vi "Begin.vi"(8 "error in":errorcluster) -> (0 "error out":errorcluster)   [LabVIEW 2020]
doc: "Called before other user functions, this VI is expected to open initial I/O refnums, load in file data, and do all program initialization. Notice that the <B>error out</B> terminal is simply used for data flow. Wiring it to other structures or subVIs ensures that this VI runs first."
uses:
  <vilib>/Rock Robotics/WPI/DriverStation/WPI_DriverStationRobotMode2.ctl
  <vilib>/Rock Robotics/WPI/Joystick/WPI_JoystickDeviceEnum.ctl
  <vilib>/Rock Robotics/WPI/SafetyOutput/WPI_SafetyOutputConfigMenu.ctl
  <vilib>/Rock Robotics/SystemInterfaces/DIO/FPGA_DIOPWMChannel.ctl
  <vilib>/Rock Robotics/WPI/RobotDrive/WPI_RobotDriveDevRef.ctl
  <vilib>/Rock Robotics/WPI/MotorControl/WPI_MotorControlDeviceRef.ctl
  <vilib>/Rock Robotics/WPI/MotorControl/WPI_MotorControlType.ctl
  <vilib>/Rock Robotics/WPI/PWM/WPI_PWMDeadband.ctl
  <vilib>/Rock Robotics/SystemInterfaces/DIO/FPGA_DIOChannel.ctl
  <vilib>/Rock Robotics/WPI/Solenoid/WPI_SolenoidChannel.ctl
  <vilib>/Rock Robotics/WPI/Compressor/WPI_CompressorFeedbackMode.ctl
  <vilib>/Rock Robotics/SystemInterfaces/spilib/spi_bus.ctl
  Robot Global Data.vi
  <vilib>/Rock Robotics/Network Tables/NT Write String Array.vi
  <vilib>/Rock Robotics/WPI/Solenoid/WPI_SolenoidOpenDouble.vi
  <vilib>/Rock Robotics/WPI/Utilities/WPI_GetSetVariantRefNum.vi
  <vilib>/Rock Robotics/WPI/MotorControl/WPI_MotorControlOpen SPARK_MAX.vi
  <vilib>/Rock Robotics/WPI/Gyro/WPI_GyroXRS450_SPI_Open.vi
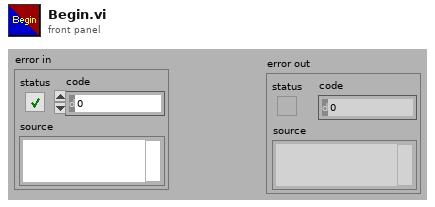
[diagram p1: front panel]
types:
  T1 = typedef "WPI_SolenoidChannel.ctl" = enum8{"Solenoid 0", "Solenoid 1", "Solenoid 2", "Solenoid 3", "Solenoid 4", "Solenoid 5", "Solenoid 6", "Solenoid 7", "Solenoid 8", "Solenoid 9", "Solenoid 10", "Solenoid 11", "Solenoid 12", "Solenoid 13", "Solenoid 14", "Solenoid 15", "Invalid"}
  T2 = typedef "spi_bus.ctl" = enum16{"SPI On-Board, CS0", "SPI On-Board, CS1", "SPI On-Board, CS2", "SPI On-Board, CS3", "SPI MXP", "Invalid"}
  T3 = typedef "WPI_CompressorFeedbackMode.ctl" = enum16{"Analog Only", "Digital Only", "Hybrid"}
  T4 = cluster{"Feedback Sensor":T3, "Max Pressure (PSI)":dbl, "Min Pressure (PSI)":dbl}
  T5 = typedef "WPI_JoystickDeviceEnum.ctl" = enum16{"USB 0", "USB 1", "USB 2", "USB 3", "USB 4", "USB 5"}
  T6 = typedef "WPI_RobotDriveDevRef.ctl" = cluster{"DevStatus":errorcluster, "Motors[]":T7[], "Square Inputs":bool, "Max Output":dbl}
  T7 = typedef "WPI_MotorControlDeviceRef.ctl" = cluster{"DeviceStatus":errorcluster, "Type":T8, "PWM":cluster{"PWM Channel":T9, "DeadBand":T10}, "CAN":cluster{"Device Number":u8, "SetOutput VI Ref":variant, "GetOutput VI Ref":variant, "Enable VI Ref":variant, "Disable VI Ref":variant, "Data":variant}, "Invert":bool, "DIO PWM":cluster{"PWM \"Enable\" Channel":T9, "DIOChannel":T11, "PWM Rate":dbl}}
  T8 = typedef "WPI_MotorControlType.ctl" = enum16{"PWM", "CAN", "DIO PWM"}
  T9 = typedef "FPGA_DIOPWMChannel.ctl" = enum8{"PWM 0", "PWM 1", "PWM 2", "PWM 3", "PWM 4", "PWM 5", "PWM 6", "PWM 7", "PWM 8", "PWM 9", "PWM MXP 0", "PWM MXP 1", "PWM MXP 2", "PWM MXP 3", "PWM MXP 4", "PWM MXP 5", "PWM MXP 6", "PWM MXP 7", "PWM MXP 8", "PWM MXP 9", "Invalid"}
  T10 = typedef "WPI_PWMDeadband.ctl" = cluster{"Name":string, "maxPositivePwm":i32, "minPositivePwm":i32, "centerPwm":i32, "maxNegativePwm":i32, "minNegativePwm":i32, "angularRange":u16}
  T11 = typedef "FPGA_DIOChannel.ctl" = enum8{"DIO 0", "DIO 1", "DIO 2", "DIO 3", "DIO 4", "DIO 5", "DIO 6", "DIO 7", "DIO 8", "DIO 9", "DIO MXP 0", "DIO MXP 1", "DIO MXP 2", "DIO MXP 3", "DIO MXP 4", "DIO MXP 5", "DIO MXP 6", "DIO MXP 7", "DIO MXP 8", "DIO MXP 9", "DIO MXP 10", "DIO MXP 11", "DIO MXP 12", "DIO MXP 13", "DIO MXP 14", "DIO MXP 15", "SPI Port CS1", "SPI Port CS2", "SPI Port CS3", "SPI Port MISO", "SPI Port MOSI", "Invalid"}
  T12 = typedef "WPI_SafetyOutputConfigMenu.ctl" = enum16{"Enable", "Disable"}
  T13 = typedef "WPI_DriverStationRobotMode2.ctl" = enum16{"Autonomous Disabled", "Autonomous Enabled", "Teleop Disabled", "Teleop Enabled", "Disconnected", "Finish", "Test Disabled", "Test Enabled", "Emergency Stopped"}
  T14 = typedef "WPI_SolenoidDevRef.ctl" = cluster{"DevStatus":errorcluster, "Pneumatics Control Module":u8, "Forward Solenoid Channel":T1, "Reverse Solenoid Channel":T1}
  T15 = typedef "WPI_JoystickDevRef.ctl" = cluster{"Device":T5}
  T16 = typedef "WPI_CompressorDevRef.ctl" = cluster{"DevStatus":errorcluster, "Pneumatics Control Module":u8}
  T17 = typedef "CTRE_Phoenix_CANcoder_DeviceRef.ctl" = cluster{"DeviceStatus":errorcluster, "Device Number":u8, "Handle":u64, "UsageFrame":u32, "Library Path":path}
  T18 = typedef "WPI_GyroDevRef.ctl" = cluster{"DevStatus":errorcluster, "Analog Channel":T19, "Gain (VoltsPerDegree/Second)":dbl, "Gyro Type":enum16{"Analog", "XRS450"}, "Handle":i32, "SPI Bus":T2, "Device Found":bool, "Sample Rate":dbl, "Calibrate On Open":bool, "Offset":dbl}
  T19 = typedef "FPGA_AIChannel.ctl" = enum8{"AI 0", "AI 1", "AI 2", "AI 3", "AI MXP 0", "AI MXP 1", "AI MXP 2", "AI MXP 3", "Invalid"}
  T20 = typedef "WPI_DigitalInputDevRef.ctl" = cluster{"DevStatus":errorcluster, "DIO Channel":T11}
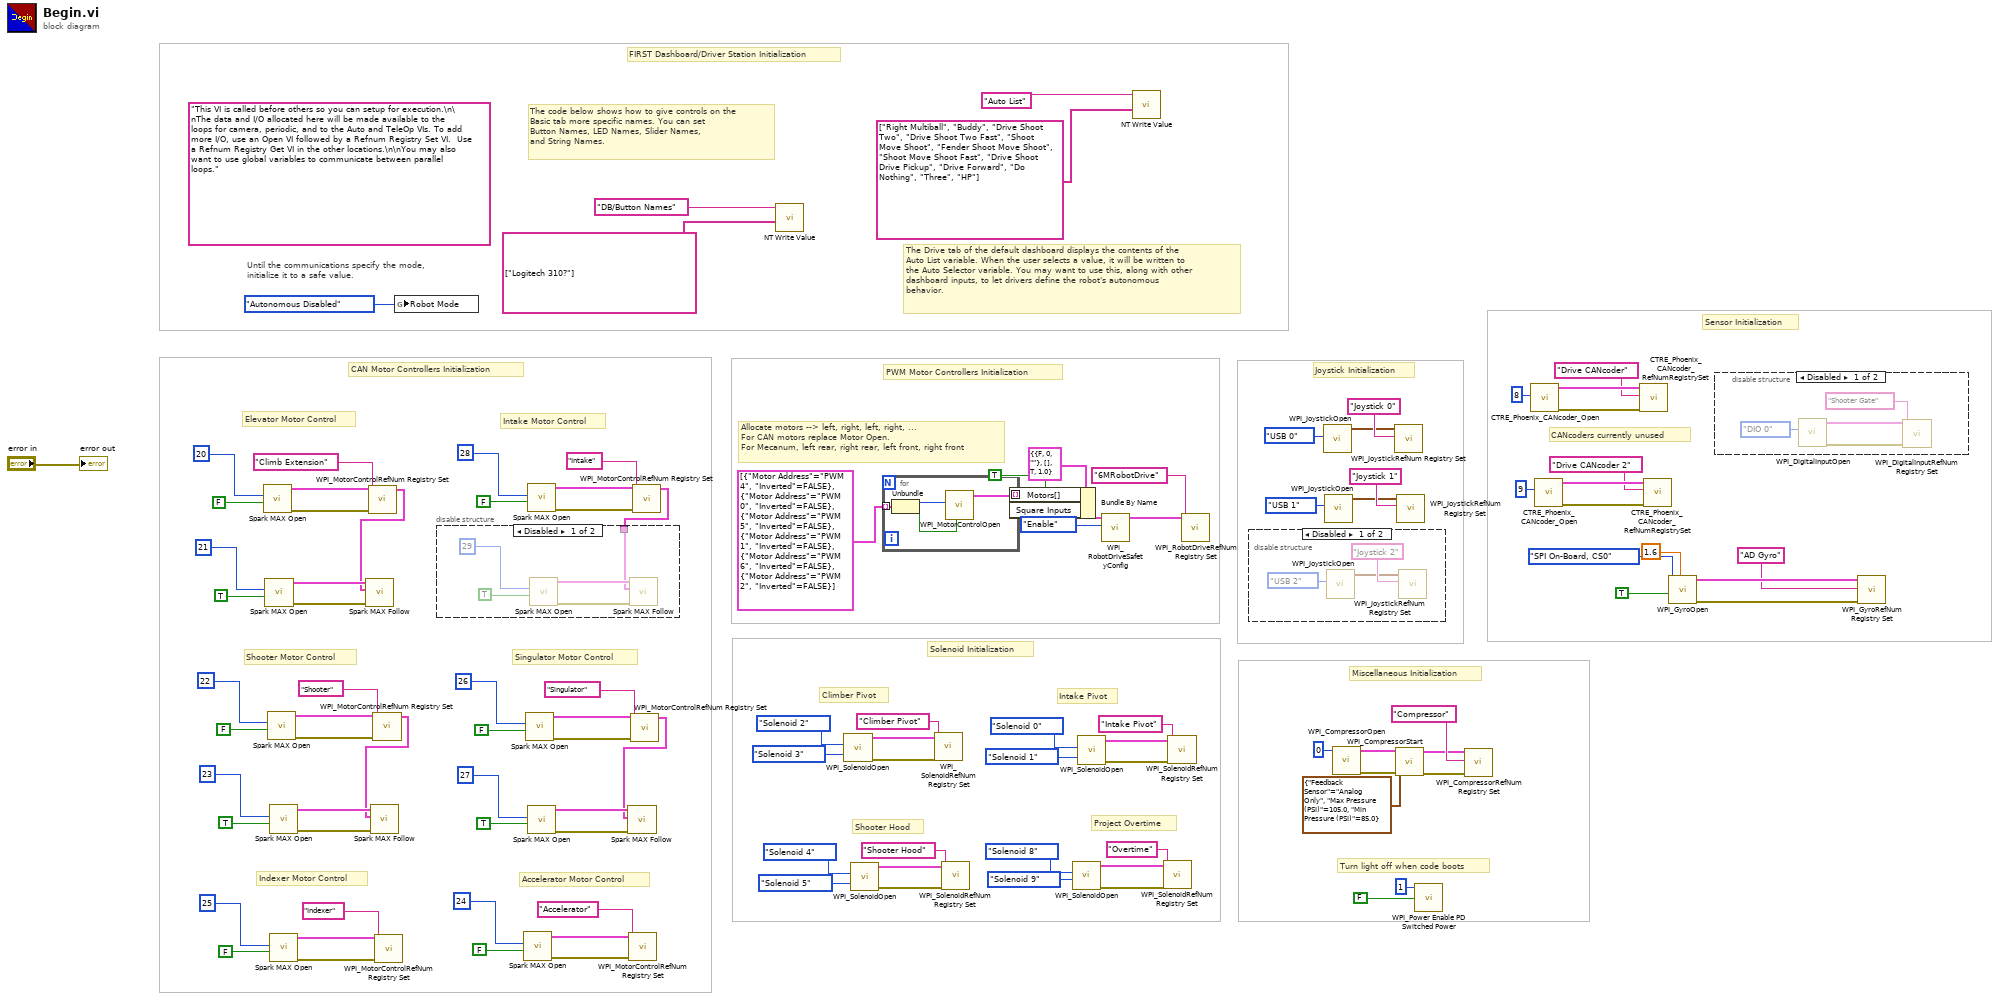
[diagram p0: block diagram]
diagram:
  (unwired) "This VI is called before others so you can setup for execution.\n\nThe data and I/O allocated here will be made available to the loops for camera, periodic, and to the Auto and TeleOp VIs. To add more I/O, use an Open VI followed by a Refnum Registry Set VI.  Use a Refnum Registry Get VI in the other locations.\n\nYou may also want to use global variables to communicate between parallel loops."
  # "Miscellaneous Initialization"
  # "Sensor Initialization"
  # "FIRST Dashboard/Driver Station Initialization"
  # "PWM Motor Controllers Initialization"
  # "Solenoid Initialization"
  # "CAN Motor Controllers Initialization"
  # "Joystick Initialization"
  # "Project Overtime"
  # "Turn light off when code boots"
  # "CANcoders currently unused"
  # "Accelerator Motor Control"
  # "Indexer Motor Control"
  # "Singulator Motor Control"
  # "Shooter Motor Control"
  # "Intake Motor Control"
  # "Shooter Hood"
  # "Intake Pivot"
  # "Climber Pivot"
  # "Elevator Motor Control"
  # "Allocate motors --> left, right, left, right, ... \nFor CAN motors replace Motor Open.\nFor Mecanum, left rear, right rear, left front, right front"
  # "The Drive tab of the default dashboard displays the contents of the\nAuto List variable. When the user selects a value, it will be written to\nthe Auto Selector variable. You may want to use this, along with other\ndashboard inputs, to let drivers define the robot's autonomous\nbehavior."
  # "The code below shows how to give controls on the\nBasic tab more specific names. You can set\nButton Names, LED Names, Slider Names,\nand String Names."
  # "Until the communications specify the mode,\ninitialize it to a safe value."
  n1 = call <vilib>:"Spark MAX Open.vi"("Invert"=FALSE, "Device Number"=u8 20) -> ("error out"=w33:errorcluster, "MotorControlDeviceRef"=w34:T7)  [unwired: 8 in]
  n2 = call <vilib>:"Spark MAX Open.vi"("Invert"=TRUE, "Device Number"=u8 21) -> ("error out"=w26:errorcluster, "MotorControlDeviceRef"=w27:T7)  [unwired: 8 in]
  n3 = call <vilib>:"Spark MAX Open.vi"("Invert"=FALSE, "Device Number"=u8 22) -> ("error out"=w49:errorcluster, "MotorControlDeviceRef"=w50:T7)  [unwired: 8 in]
  n4 = call <vilib>:"Spark MAX Open.vi"("Invert"=TRUE, "Device Number"=u8 23) -> ("error out"=w42:errorcluster, "MotorControlDeviceRef"=w43:T7)  [unwired: 8 in]
  n5 = call <vilib>:"Spark MAX Open.vi"("Invert"=FALSE, "Device Number"=u8 25) -> ("error out"=w62:errorcluster, "MotorControlDeviceRef"=w63:T7)  [unwired: 8 in]
  n6 = call <vilib>:"WPI_MotorControlRefNum Registry Set.vi"("error in (no error)"=w33, "refnum name"="Climb Extension", "MotorControlDevRef"=w34) -> ("MotorControlDevRef"=w25:T7)  [unwired: 7 in, 1 out]
  n7 = call <vilib>:"Spark MAX Follow.vi"("error in (no error)"=w26, "Master Controller"=w25, "MotorControlDeviceRef"=w27) -> ()  [unwired: 7 in, 2 out]
  n8 = call <vilib>:"WPI_MotorControlRefNum Registry Set.vi"("error in (no error)"=w49, "refnum name"="Shooter", "MotorControlDevRef"=w50) -> ("MotorControlDevRef"=w41:T7)  [unwired: 7 in, 1 out]
  n9 = call <vilib>:"Spark MAX Follow.vi"("error in (no error)"=w42, "Master Controller"=w41, "MotorControlDeviceRef"=w43) -> ()  [unwired: 7 in, 2 out]
  n10 = call <vilib>:"WPI_MotorControlRefNum Registry Set.vi"("error in (no error)"=w62, "refnum name"="Indexer", "MotorControlDevRef"=w63) -> ()  [unwired: 7 in, 2 out]
  n11 = global write "Robot Global Data.vi" "Robot Mode"(WPI_DriverStationRobotMode2."Autonomous Disabled" ("Robot Mode")) -> ()
  n12 = call <vilib>:"Spark MAX Open.vi"("Invert"=FALSE, "Device Number"=u8 24) -> ("error out"=w57:errorcluster, "MotorControlDeviceRef"=w58:T7)  [unwired: 8 in]
  n13 = call <vilib>:"Spark MAX Open.vi"("Invert"=FALSE, "Device Number"=u8 26) -> ("error out"=w69:errorcluster, "MotorControlDeviceRef"=w70:T7)  [unwired: 8 in]
  n14 = call <vilib>:"Spark MAX Open.vi"("Invert"=FALSE, "Device Number"=u8 28) -> ("error out"=w39:errorcluster, "MotorControlDeviceRef"=w40:T7)  [unwired: 8 in]
  n15 = call <vilib>:"Spark MAX Open.vi"("Invert"=TRUE, "Device Number"=u8 27) -> ("error out"=w52:errorcluster, "MotorControlDeviceRef"=w53:T7)  [unwired: 8 in]
  n16 = call <vilib>:"WPI_MotorControlRefNum Registry Set.vi"("error in (no error)"=w57, "refnum name"="Accelerator", "MotorControlDevRef"=w58) -> ()  [unwired: 7 in, 2 out]
  n17 = call <vilib>:"WPI_MotorControlRefNum Registry Set.vi"("error in (no error)"=w69, "refnum name"="Singulator", "MotorControlDevRef"=w70) -> ("MotorControlDevRef"=w51:T7)  [unwired: 7 in, 1 out]
  n18 = call <vilib>:"Spark MAX Follow.vi"("error in (no error)"=w52, "Master Controller"=w51, "MotorControlDeviceRef"=w53) -> ()  [unwired: 7 in, 2 out]
  n19 = call <vilib>:"WPI_MotorControlRefNum Registry Set.vi"("error in (no error)"=w39, "refnum name"="Intake", "MotorControlDevRef"=w40) -> ("MotorControlDevRef"=w35:T7)  [unwired: 7 in, 1 out]
  n20 = disable-structure shown="Disabled" {
    disable-tunnel: w35 -> [w110 _]
    frame Disabled {
      n21 = call <vilib>:"Spark MAX Open.vi"("Invert"=TRUE, "Device Number"=u8 29) -> ("error out"=w111:errorcluster, "MotorControlDeviceRef"=w112:T7)  [unwired: 8 in]
      n22 = call <vilib>:"Spark MAX Follow.vi"("error in (no error)"=w111, "Master Controller"=w110, "MotorControlDeviceRef"=w112) -> ()  [unwired: 7 in, 2 out]
    }
    frame Enabled {
    }
  }
  n23 = call-poly <vilib>:"NT Write Value.vi"("String Array"=string[] ["Logitech 310?"], "Name"="DB/Button Names") -> ()  [unwired: 9 in, 1 out]
  n24 = call-poly <vilib>:"WPI_SolenoidOpen.vi"("Reverse Solenoid Channel"=WPI_SolenoidChannel."Solenoid 3", "Forward Solenoid Channel"=WPI_SolenoidChannel."Solenoid 2") -> ("error out"=w84:errorcluster, "SolenoidDevRef"=w85:T14)  [unwired: 8 in]
  n25 = call-poly <vilib>:"WPI_SolenoidOpen.vi"("Reverse Solenoid Channel"=WPI_SolenoidChannel."Solenoid 5", "Forward Solenoid Channel"=WPI_SolenoidChannel."Solenoid 4") -> ("error out"=w79:errorcluster, "SolenoidDevRef"=w80:T14)  [unwired: 8 in]
  n26 = for {
    tunnel: cluster{"Motor Address":T9, "Inverted":bool}[] [{"Motor Address"=enum."PWM 4", "Inverted"=FALSE}, {"Motor Address"=enum."PWM 0", "Inverted"=FALSE}, {"Motor Address"=enum."PWM 5", "Inverted"=FALSE}, {"Motor Address"=enum."PWM 1", "Inverted"=FALSE}, {"Motor Address"=enum."PWM 6", "Inverted"=FALSE}, {"Motor Address"=enum."PWM 2", "Inverted"=FALSE}] ("Array") -> [w118] mode=indexing
    tunnel: [w115] -> w100 mode=indexing
    n27 = Unbundle(w118) -> ("Motor Address"=w117:T9, "Inverted"=w116:bool)
    n28 = call-poly <vilib>:"WPI_MotorControlOpen.vi"("Invert"=w116, "PWM Channel"=w117) -> ("MotorControlDeviceRef"=w115:T7)  [unwired: 2 in, 7 out]
  }
  n29 = call <vilib>:"WPI_SolenoidRefNum Registry Set.vi"("error in (no error)"=w84, "refnum name"="Climber Pivot", "SolenoidDevRef"=w85) -> ()  [unwired: 7 in, 2 out]
  n30 = call <vilib>:"WPI_SolenoidRefNum Registry Set.vi"("error in (no error)"=w79, "refnum name"="Shooter Hood", "SolenoidDevRef"=w80) -> ()  [unwired: 7 in, 2 out]
  n31 = Bundle By Name(cluster=T6 {"DevStatus"={"status"=FALSE, "code"=0, "source"=""}, "Motors[]"=[], "Square Inputs"=TRUE, "Max Output"=1.0} ("RobotDriveDevRef"), "Motors[]"=w100, "Square Inputs"=TRUE) -> (w98:T6)
  n32 = call-poly <vilib>:"WPI_SolenoidOpen.vi"("Reverse Solenoid Channel"=WPI_SolenoidChannel."Solenoid 9", "Forward Solenoid Channel"=WPI_SolenoidChannel."Solenoid 8") -> ("error out"=w4:errorcluster, "SolenoidDevRef"=w5:T14)  [unwired: 8 in]
  n33 = call-poly <vilib>:"WPI_SolenoidOpen.vi"("Reverse Solenoid Channel"=WPI_SolenoidChannel."Solenoid 1", "Forward Solenoid Channel"=WPI_SolenoidChannel."Solenoid 0") -> ("error out"=w89:errorcluster, "SolenoidDevRef"=w90:T14)  [unwired: 8 in]
  n34 = call <vilib>:"WPI_RobotDriveSafetyConfig.vi"("mode"=WPI_SafetyOutputConfigMenu."Enable", "RobotDriveDevRef"=w98) -> ("RobotDriveDevRef"=w95:T6)  [unwired: 2 in, 7 out]
  n35 = call-poly <vilib>:"NT Write Value.vi"("String Array"=string[] ["Right Multiball", "Buddy", "Drive Shoot Two", "Drive Shoot Two Fast", "Shoot Move Shoot", "Fender Shoot Move Shoot", "Shoot Move Shoot Fast", "Drive Shoot Drive Pickup", "Drive Forward", "Do Nothing", "Three", "HP"], "Name"="Auto List") -> ()  [unwired: 9 in, 1 out]
  n36 = call <vilib>:"WPI_SolenoidRefNum Registry Set.vi"("error in (no error)"=w4, "refnum name"="Overtime", "SolenoidDevRef"=w5) -> ()  [unwired: 7 in, 2 out]
  n37 = call <vilib>:"WPI_SolenoidRefNum Registry Set.vi"("error in (no error)"=w89, "refnum name"="Intake Pivot", "SolenoidDevRef"=w90) -> ()  [unwired: 7 in, 2 out]
  n38 = call <vilib>:"WPI_RobotDriveRefNum Registry Set.vi"("refnum name"="6MRobotDrive", "RobotDriveDevRef"=w95) -> ()  [unwired: 8 in, 2 out]
  n39 = disable-structure shown="Disabled" {
    frame Disabled {
      n40 = call <vilib>:"WPI_JoystickOpen.vi"("JoystickDevice"=WPI_JoystickDeviceEnum."USB 2") -> ("JoystickDevRef"=w120:T15)  [unwired: 10 in]
      n41 = call <vilib>:"WPI_JoystickRefNum Registry Set.vi"("refnum name"="Joystick 2", "JoystickDevRef"=w120) -> ()  [unwired: 8 in, 2 out]
    }
    frame Enabled {
    }
  }
  n42 = call <vilib>:"WPI_JoystickOpen.vi"("JoystickDevice"=WPI_JoystickDeviceEnum."USB 0") -> ("JoystickDevRef"=w107:T15)  [unwired: 10 in]
  n43 = call <vilib>:"WPI_JoystickOpen.vi"("JoystickDevice"=WPI_JoystickDeviceEnum."USB 1") -> ("JoystickDevRef"=w92:T15)  [unwired: 10 in]
  n44 = call <vilib>:"WPI_CompressorOpen.vi"("Pneumatics device (def)"=u8 0) -> ("CompressorDevRef"=w74:T16, "error out"=w72:errorcluster)  [unwired: 13 in]
  n45 = call <vilib>:"WPI_JoystickRefNum Registry Set.vi"("refnum name"="Joystick 0", "JoystickDevRef"=w107) -> ()  [unwired: 8 in, 2 out]
  n46 = call <vilib>:"WPI_CompressorStart.vi"("error in (no error)"=w72, "Feedback Configuration"=T4 {"Feedback Sensor"=enum."Analog Only", "Max Pressure (PSI)"=105.0, "Min Pressure (PSI)"=85.0}, "CompressorDevRef"=w74) -> ("error out"=w71:errorcluster, "CompressorDevRef"=w73:T16)  [unwired: 7 in]
  n47 = call <vilib>:"WPI_JoystickRefNum Registry Set.vi"("refnum name"="Joystick 1", "JoystickDevRef"=w92) -> ()  [unwired: 8 in, 2 out]
  n48 = call <vilib>:"WPI_Power Enable PD Switched Power.vi"("Power Distribution (def)"=u8 1, "Switch Channel Value"=FALSE) -> ()  [unwired: 12 in, 2 out]
  n49 = call <vilib>:"WPI_CompressorRefNum Registry Set.vi"("error in (no error)"=w71, "refnum name"="Compressor", "CompressorDevRef"=w73) -> ()  [unwired: 7 in, 2 out]
  n50 = call <vilib>:"CTRE_Phoenix_CANcoder_Open.vi"("Device Number"=u8 8) -> ("error out"=w20:errorcluster, "CTRE_CANcoder_DeviceRef"=w21:T17)  [unwired: 9 in]
  n51 = call <vilib>:"CTRE_Phoenix_CANcoder_Open.vi"("Device Number"=u8 9) -> ("error out"=w16:errorcluster, "CTRE_CANcoder_DeviceRef"=w17:T17)  [unwired: 9 in]
  n52 = call <vilib>:"CTRE_Phoenix_CANcoder_RefNumRegistrySet.vi"("error in (no error)"=w20, "refnum name"="Drive CANcoder", "CTRE_CANcoder_DeviceRef"=w21) -> ()  [unwired: 7 in, 2 out]
  n53 = call <vilib>:"CTRE_Phoenix_CANcoder_RefNumRegistrySet.vi"("error in (no error)"=w16, "refnum name"="Drive CANcoder 2", "CTRE_CANcoder_DeviceRef"=w17) -> ()  [unwired: 7 in, 2 out]
  n54 = call-poly <vilib>:"WPI_GyroOpen.vi"("Calibration Time (s)"=1.6, "Calibrate On Open"=TRUE, "SPI Bus"=spi_bus."SPI On-Board, CS0") -> ("error out"=w9:errorcluster, "GyroDevRef"=w13:T18)  [unwired: 6 in, 1 out]
  n55 = disable-structure shown="Disabled" {
    frame Disabled {
      n56 = call <vilib>:"WPI_DigitalInputOpen.vi"("DIO Channel"=FPGA_DIOChannel."DIO 0") -> ("error out"=w123:errorcluster, "DigitalInputDevRef"=w125:T20)  [unwired: 9 in]
      n57 = call <vilib>:"WPI_DigitalInputRefNum Registry Set.vi"("error in (no error)"=w123, "refnum name"="Shooter Gate", "DigitalInputDevRef"=w125) -> ()  [unwired: 7 in, 2 out]
    }
    frame Enabled {
    }
  }
  n58 = call <vilib>:"WPI_GyroRefNum Registry Set.vi"("error in (no error)"=w9, "refnum name"="AD Gyro", "GyroDevRef"=w13) -> ()  [unwired: 7 in, 2 out]
  "error out" <- "error in"
